vi "PopulateRingObj.vi"(0 "Data []":cluster{"Description":string, "Code":u8}[](array[cluster]), 2 "error in (no error)":errorcluster, 12 "reference":refnum<vi>) -> (22 "error out":errorcluster)   [LabVIEW 2020, in "CameraTestingUI.lvlib" / "CameraTestingUI.lvclass"]
uses:
  CameraTestingUI.lvclass
  CameraTestingUI.lvclass/CameraTestingUI.ctl
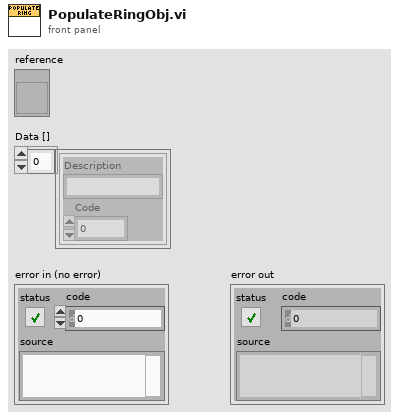
[diagram p1: front panel]
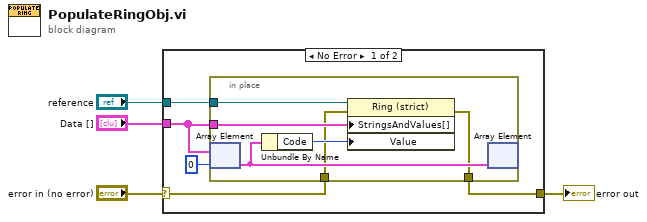
[diagram p0: block diagram]
diagram:
  n1 = case shown="No Error" "error in (no error)" {
    selector: "error in (no error)" -> [w6 w16]
    tunnel: "reference" -> [w7 _]
    tunnel: "Data []" -> [w8 _]
    tunnel: [w5 w16] -> w2
    frame No Error {
      n2 = in-place {
        in-place-border: w8 -> [w13]
        in-place-border: w7 -> [w12]
        in-place-border: w6 -> [w11]
        in-place-border: [w10] -> w5
        n3 = in-place-array #1(w8, 0) -> (w14:cluster{"Description":string, "Code":u8})
        n4 = Unbundle By Name(w14) -> ("Code"=w15:u8)
        n5 = property on="Property Node" class="Ring (strict)"(reference=w12, error in=w11, "StringsAndValues[]"=w13, "Value"=w15) -> (error out=w10:errorcluster)  [unwired: 1 out]
        n6 = in-place-array #1(w14) -> ()  [unwired: 2 out]
      }
    }
    frame Error {
    }
  }
  "error out" <- w2
